vi "_PC_Err get_err_call_chain.vi"() -> (0 "call chain string":string)   [LabVIEW 2018]
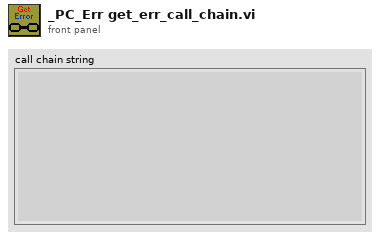
[diagram p1: front panel]
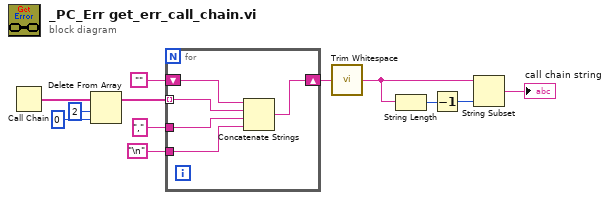
[diagram p0: block diagram]
diagram:
  n1 = Call Chain() -> (call chain=w10:string[])
  n2 = Delete From Array(array=w10, length=2, index=0) -> (array with subset deleted=w9:string[])  [unwired: 1 out]
  n3 = for {
    tunnel: w9 -> [w17] mode=indexing
    shift-right: [w15] -> w7
    shift-left: "" -> [w16]
    tunnel: "," -> [w14]
    tunnel: "\n" -> [w13]
    n4 = Concatenate Strings(w16, w17, w14, w13) -> (w15:string)
  }
  n5 = call <vilib>:"Trim Whitespace.vi"("string"=w7) -> ("trimmed string"=w4:string)  [unwired: 1 in]
  n6 = String Length(string=w4) -> (length=w3:i32)
  n7 = Decrement(x=w3) -> (x-1=w2:i32)
  n8 = String Subset(string=w4, length (rest)=w2) -> (substring=→"call chain string":string)  [unwired: 1 in]
